vi "Image Display Get Pixel Color Information.vi"(5 "Image High Color":u32(colorbox)=16777216, 7 "Image Low Color":u32(colorbox)=16777216, 8 "Error In":errorcluster, 10 "Image Display Range":cluster{"Min Value":sgl, "Max Value":sgl}={"Min Value"=nan, "Max Value"=nan}, 11 "Image Display Palette Information":T1 {"Palette Type" items=["Grayscale", "Binary", "Gradient", "Rainbow", "Temperature", "User Defined", "Binary 16 Bit", "Gradient 16 Bit", "Rainbow 16 Bit", "Temperature 16 Bit", "User Defined 16 Bit"]}) -> (0 "Error Out":errorcluster, 1 "Image Scale Factor (256 colors)":sgl, 2 "Image Range Min Value":sgl, 3 "1D Color Array":cluster{"Red":u8, "Green":u8, "Blue":u8}[](array[cluster]))   [LabVIEW 2021, in "Palette.lvlib"]
doc: "Provide the <B>Image Display Range</B> and <B>Image Display Palette Information</B> when first calling this VI (setting <B>Init Palette</B> = TRUE), and if appropriate, the <B>Image High Color</B> and <B>Image Low Color</B> parameters."
uses:
  Palette/Palette.lvlib
  Palette/Image Palette Information.ctl
  Image Display Palette Type.ctl
  Image.lvlib
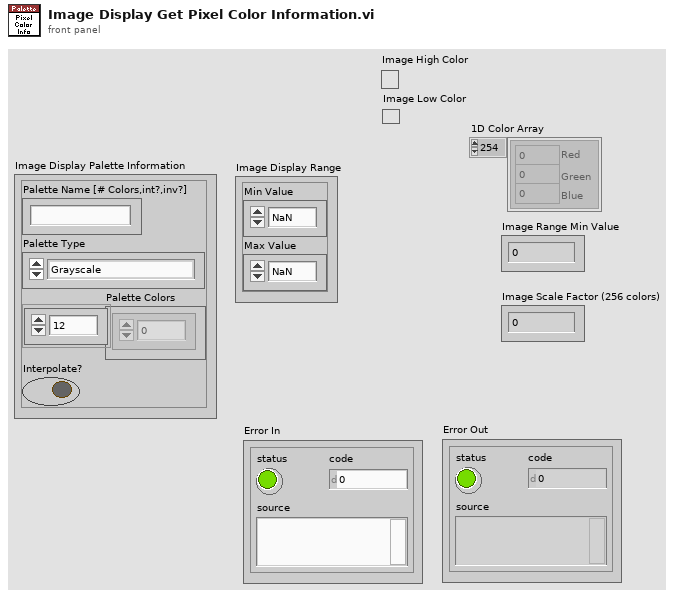
[diagram p1: front panel]
types:
  T1 = typedef "Palette.lvlib/Image Palette Information.ctl" = cluster{"Palette Name [# Colors,int?,inv?]":string, "Palette Type":T2, "Palette Colors":u32[], "Interpolate?":bool}
  T2 = typedef "Image.lvlib/Image Display Palette Type.ctl" = u32
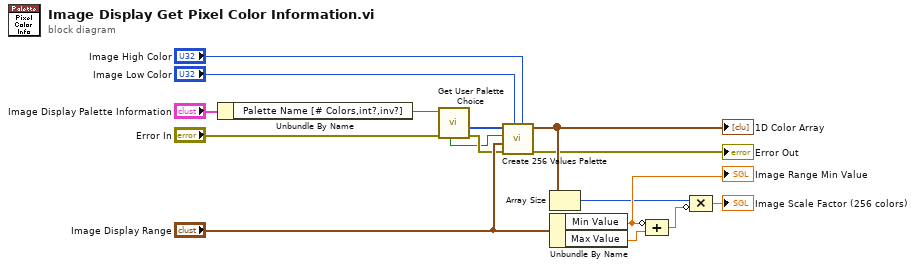
[diagram p0: block diagram]
diagram:
  n1 = Unbundle By Name("Image Display Palette Information") -> ("Palette Name [# Colors,int?,inv?]"=w8:string)
  n2 = call "Get User Palette Choice.vi"("Error In"="Error In", "Palette"=w8) -> ("Error Out"=w6:errorcluster, "Palette Colors"=w7:u32[], "Interpolate?"=w1:bool)  [unwired: 2 in, 5 out]
  n3 = call "Create 256 Values Palette.vi"("Image High Color"="Image High Color", "Image Low Color"="Image Low Color", "Error In"=w6, "Source Image Display Range"="Image Display Range", "Interpolate?"=w1, "Palette Colors in"=w7) -> ("Error Out"=→"Error Out":errorcluster, "1D Color value array"=w10:cluster{"Red":u8, "Green":u8, "Blue":u8}[])  [unwired: 2 in, 2 out]
  "1D Color Array" <- w10
  n4 = Array Size(array=w10) -> (size(s)=w2:i32)
  n5 = Unbundle By Name("Image Display Range") -> ("Min Value"=w5:sgl, "Max Value"=w4:sgl)
  "Image Range Min Value" <- w5
  n6 = Compound Arithmetic op=ADD(invert w5, w4) -> (w3:sgl)
  n7 = Compound Arithmetic op=MULTIPLY(w2, invert w3) -> (→"Image Scale Factor (256 colors)":sgl)
